vi "Open_Instr.vi"(8 "error in (no error)":errorcluster caption="entrée d'erreur (pas d'erreur)", 11 "Class Multimeter (Default) en entrée":refnum<class "Class Instrument Process.lvclass">) -> (0 "error out":errorcluster caption="sortie d'erreur", 3 "Class Multimeter (Default) en sortie":refnum<class "Class Instrument Process.lvclass">)   [LabVIEW 2020, in "Library Instrument & Equipement.lvlib" / "Library Instruments.lvlib" / "Class Instrument Process.lvclass"]
doc: "Opens and acquires an instrument"
uses:
  Class Instrument Process.lvclass
  Class Instrument Process.lvclass/Class Instrument Process.ctl
  Instrument (Default)/Class Instrument (Default).lvclass
  Process/Process (Default)/Process (Default).lvclass
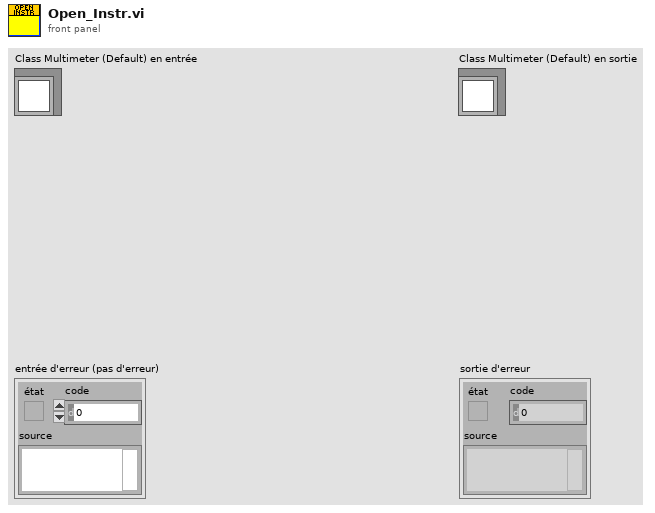
[diagram p1: front panel]
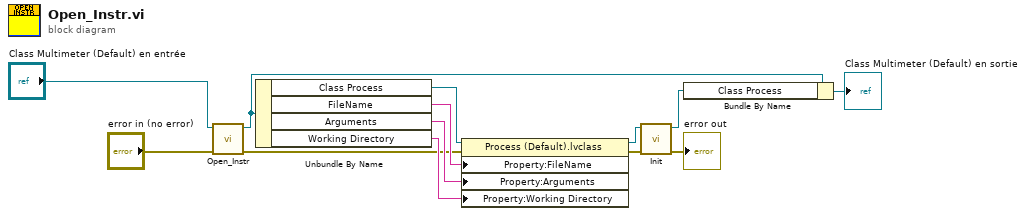
[diagram p0: block diagram]
diagram:
  n1 = call-parent "Open_Instr.vi"("error in (no error)"="error in (no error)", "Class Multimeter (Default) en entrée"="Class Multimeter (Default) en entrée") -> ("error out"=w3:errorcluster, "Class Multimeter (Default) en sortie"=w4:refnum<class "Class Instrument Process.lvclass">)  [unwired: 8 in]
  n2 = Unbundle By Name(w4) -> ("Class Process"=w10:refnum<class "Process (Default).lvclass">, "FileName"=w9:string, "Arguments"=w8:string, "Working Directory"=w7:string)
  n3 = property class="Process (Default).lvclass"(reference=w10, error in=w3, "Property:FileName"=w9, "Property:Arguments"=w8, "Property:Working Directory"=w7) -> (reference out=w5:refnum<class "Process (Default).lvclass">, error out=w6:errorcluster)
  n4 = call-dynamic "Init.vi"("error in (no error)"=w6, "Process (Default) en entrée"=w5) -> ("error out"=→"error out":errorcluster, "Process (Default) en sortie"=w1:refnum<class "Process (Default).lvclass">)  [unwired: 8 in]
  n5 = Bundle By Name(cluster=w4, "Class Process"=w1) -> (→"Class Multimeter (Default) en sortie":refnum<class "Class Instrument Process.lvclass">)
